vi "Drop Messages.vi"(8 "error in":errorcluster, 10 "Drop?":bool=TRUE, 11 "log in":T1) -> (0 "error out":errorcluster, 2 "Current Msgs":string[](array[string]), 3 "log out":T1)   [LabVIEW 2016, in "System Log.lvclass"]
doc: "Drop all messages in the current message queue."
uses:
  System Log.lvclass
  _Session Fwk/Typedefs/Session Handle.ctl
  _Session Fwk/Session - Root.lvclass
  G:/sw_repo/For Builds/Reusable/Session APIs/_Session Fwk/Session - Root.lvclass
  System Log.lvclass/System Log.ctl
  Accessors/Write Current Message.vi
  Accessors/Read Current Message.vi
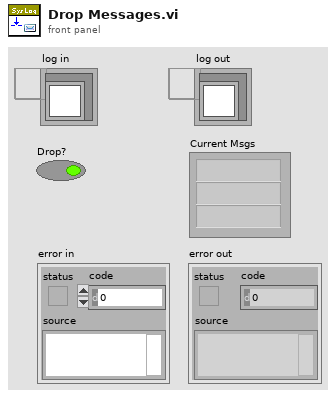
[diagram p1: front panel]
types:
  T1 = typedef "Session - Root.lvclass/Session Handle.ctl" = refnum<data-value>
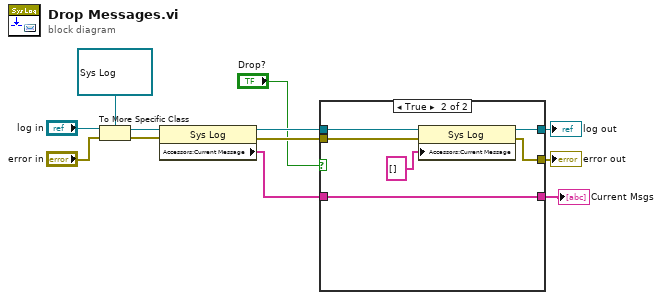
[diagram p0: block diagram]
diagram:
  n1 = To More Specific Class(target class=refnum<data-value> refnum ("log"), reference="log in", error in="error in") -> (specific class reference=w1:refnum<data-value>, error out=w6:errorcluster)
  n2 = property class="Sys Log"(reference=w1, error in=w6) -> (reference out=w10:refnum<data-value>, error out=w5:errorcluster, "Accessors:Current Message"=w2:string[])
  n3 = case shown="True" "Drop?" {
    tunnel: w10 -> [w15 w21]
    tunnel: [w15 w20] -> w9
    tunnel: [w14 w19] -> w8
    tunnel: w5 -> [w14 w18]
    tunnel: w2 -> [w13 w16]
    tunnel: [w13 w16] -> w3
    frame False {
    }
    frame True {
      n4 = property class="Sys Log"(reference=w21, error in=w18, "Accessors:Current Message"=string[] [] ("Current Msgs")) -> (reference out=w20:refnum<data-value>, error out=w19:errorcluster)
    }
  }
  "error out" <- w8
  "Current Msgs" <- w3
  "log out" <- w9
